vi "globalprogram.vi"() -> (2 "Array 2":i32[](array[numeric]), 3 "Numeric 2":i32)   [LabVIEW 2019]
uses:
  <vilib>/myRIO/Common/Instrument Driver Framework/Utilities/typedefs/Analog Scaling Constants.ctl
  <vilib>/myRIO/Common/Instrument Driver Framework/Utilities/typedefs/Analog Scaling Constants List.ctl
  <vilib>/myRIO/Common/Instrument Driver Framework/myRIO v1.0/AO/typedefs/AO Channels Enum.ctl
  <vilib>/myRIO/Common/Instrument Driver Framework/myRIO v1.0/AO/typedefs/AO Channels List.ctl
  <vilib>/myRIO/Common/Instrument Driver Framework/Utilities/typedefs/Generic FPGA Reference.ctl
  <vilib>/myRIO/Common/Instrument Driver Framework/Utilities/typedefs/myRIO v1.0 Reference.ctl
  <vilib>/myRIO/Common/Instrument Driver Framework/Utilities/typedefs/Hardware Version Enum.ctl
  <vilib>/myRIO/Common/Instrument Driver Framework/Utilities/typedefs/myRIO Generic Hardware Reference.ctl
  <vilib>/myRIO/Instrument Drivers/Onboard IO/AO/typedefs/AO Reference.ctl
  <vilib>/myRIO/Instrument Drivers/Onboard IO/AO/AO.lvlib
  <vilib>/myRIO/Instrument Drivers/Onboard IO/AO/vis/Write.vi
  <vilib>/userDefined/High Color/nirio_resource_hc.ctl
  <vilib>/myRIO/Common/Instrument Driver Framework/myRIO v1.0/AO/vis/myRIO v1.1 Open AO.vi
  <vilib>/myRIO/Instrument Drivers/Onboard IO/AO/vis/myRIO AO Open.xnode
  <vilib>/myRIO/Common/Instrument Driver Framework/Utilities/vis/Is FPGA Ref Available.vi
  <vilib>/myRIO/Express VI/Onboard IO/AO/AO Express VI.xnode
  Global 1.vi
  <vilib>/myRIO/Common/Instrument Driver Framework/myRIO v1.0/AI/typedefs/AI Channels Enum.ctl
  <vilib>/myRIO/Common/Instrument Driver Framework/myRIO v1.0/AI/typedefs/AI Channels List.ctl
  <vilib>/myRIO/Instrument Drivers/Onboard IO/AI/typedefs/AI Reference.ctl
  <vilib>/myRIO/Instrument Drivers/Onboard IO/AI/AI.lvlib
  <vilib>/myRIO/Instrument Drivers/Onboard IO/AI/vis/Read.vi
  <vilib>/myRIO/Common/Instrument Driver Framework/myRIO v1.0/AI/vis/myRIO v1.1 Open AI.vi
  <vilib>/myRIO/Instrument Drivers/Onboard IO/AI/vis/myRIO AI Open.xnode
  <vilib>/myRIO/Express VI/Onboard IO/AI/AI Express VI.xnode
  <vilib>/myRIO/Express VI/Onboard IO/DI/DI Express VI.xnode
  <vilib>/myRIO/Instrument Drivers/Onboard IO/DIO/vis/Read.vi
  <vilib>/myRIO/Instrument Drivers/Onboard IO/DIO/DIO.lvlib
  <vilib>/myRIO/Common/Instrument Driver Framework/myRIO v1.0/DIO/typedefs/DIO Channels Enum.ctl
  <vilib>/myRIO/Common/Instrument Driver Framework/myRIO v1.0/DIO/typedefs/DIO Channels List.ctl
  <vilib>/myRIO/Instrument Drivers/Onboard IO/DIO/typedefs/DIO Reference.ctl
  <vilib>/myRIO/Instrument Drivers/Onboard IO/DIO/vis/myRIO DIO Open.xnode
  <vilib>/myRIO/Instrument Drivers/Onboard IO/I2C/typedefs/I2C Transfer Rate.ctl
  <vilib>/myRIO/Instrument Drivers/Onboard IO/I2C/I2C.lvlib
  <vilib>/myRIO/Instrument Drivers/Onboard IO/I2C/typedefs/I2C User Configuration.ctl
  <vilib>/myRIO/Instrument Drivers/Onboard IO/I2C/typedefs/I2C Configuration.ctl
  <vilib>/myRIO/Common/Instrument Driver Framework/myRIO v1.0/I2C/typedefs/I2C Channels Enum.ctl
  <vilib>/myRIO/Instrument Drivers/Onboard IO/I2C/typedefs/I2C Reference.ctl
  <vilib>/myRIO/Instrument Drivers/Onboard IO/I2C/vis/Configure.vi
  <vilib>/myRIO/Instrument Drivers/Onboard IO/I2C/vis/Write.vi
  <vilib>/myRIO/Common/Instrument Driver Framework/myRIO v1.0/I2C/vis/myRIO v1.1 Open I2C.vi
  <vilib>/myRIO/Instrument Drivers/Onboard IO/I2C/vis/myRIO I2C Open.xnode
  <vilib>/myRIO/Express VI/Onboard IO/I2C/I2C Express VI.xnode
  <vilib>/myRIO/Common/Instrument Driver Framework/myRIO v1.0/DIO/vis/myRIO v1.1 Open DIO.vi
panel:
  in  "tijdsinterval 8":dbl
  in  "tijdsinterval 7":dbl
  in  "tijdsinterval 6":dbl
  in  "tijdsinterval 5":dbl
  in  "tijdsinterval 4":dbl
  in  "tijdsinterval 3":dbl
  in  "tijdsinterval 2":dbl
  out "groen":u32
  out "rood":u32
  out "error out 3":errorcluster
  in  "error in (no error) 3":errorcluster
  out "A/DIO1 (Pin 13)":bool
  in  "stoppen":bool
  in  "rechts draaien achteruit":bool
  in  "links draaien achteruit":bool
  out "appended array":dbl[](array[numeric])
  in  "snelheid":dbl
  in  "rechts draaien":bool
  in  "links draaien":bool
  in  "achterwaarts":bool
  in  "voorwaarts":bool
  in  "Boolean manueel":bool
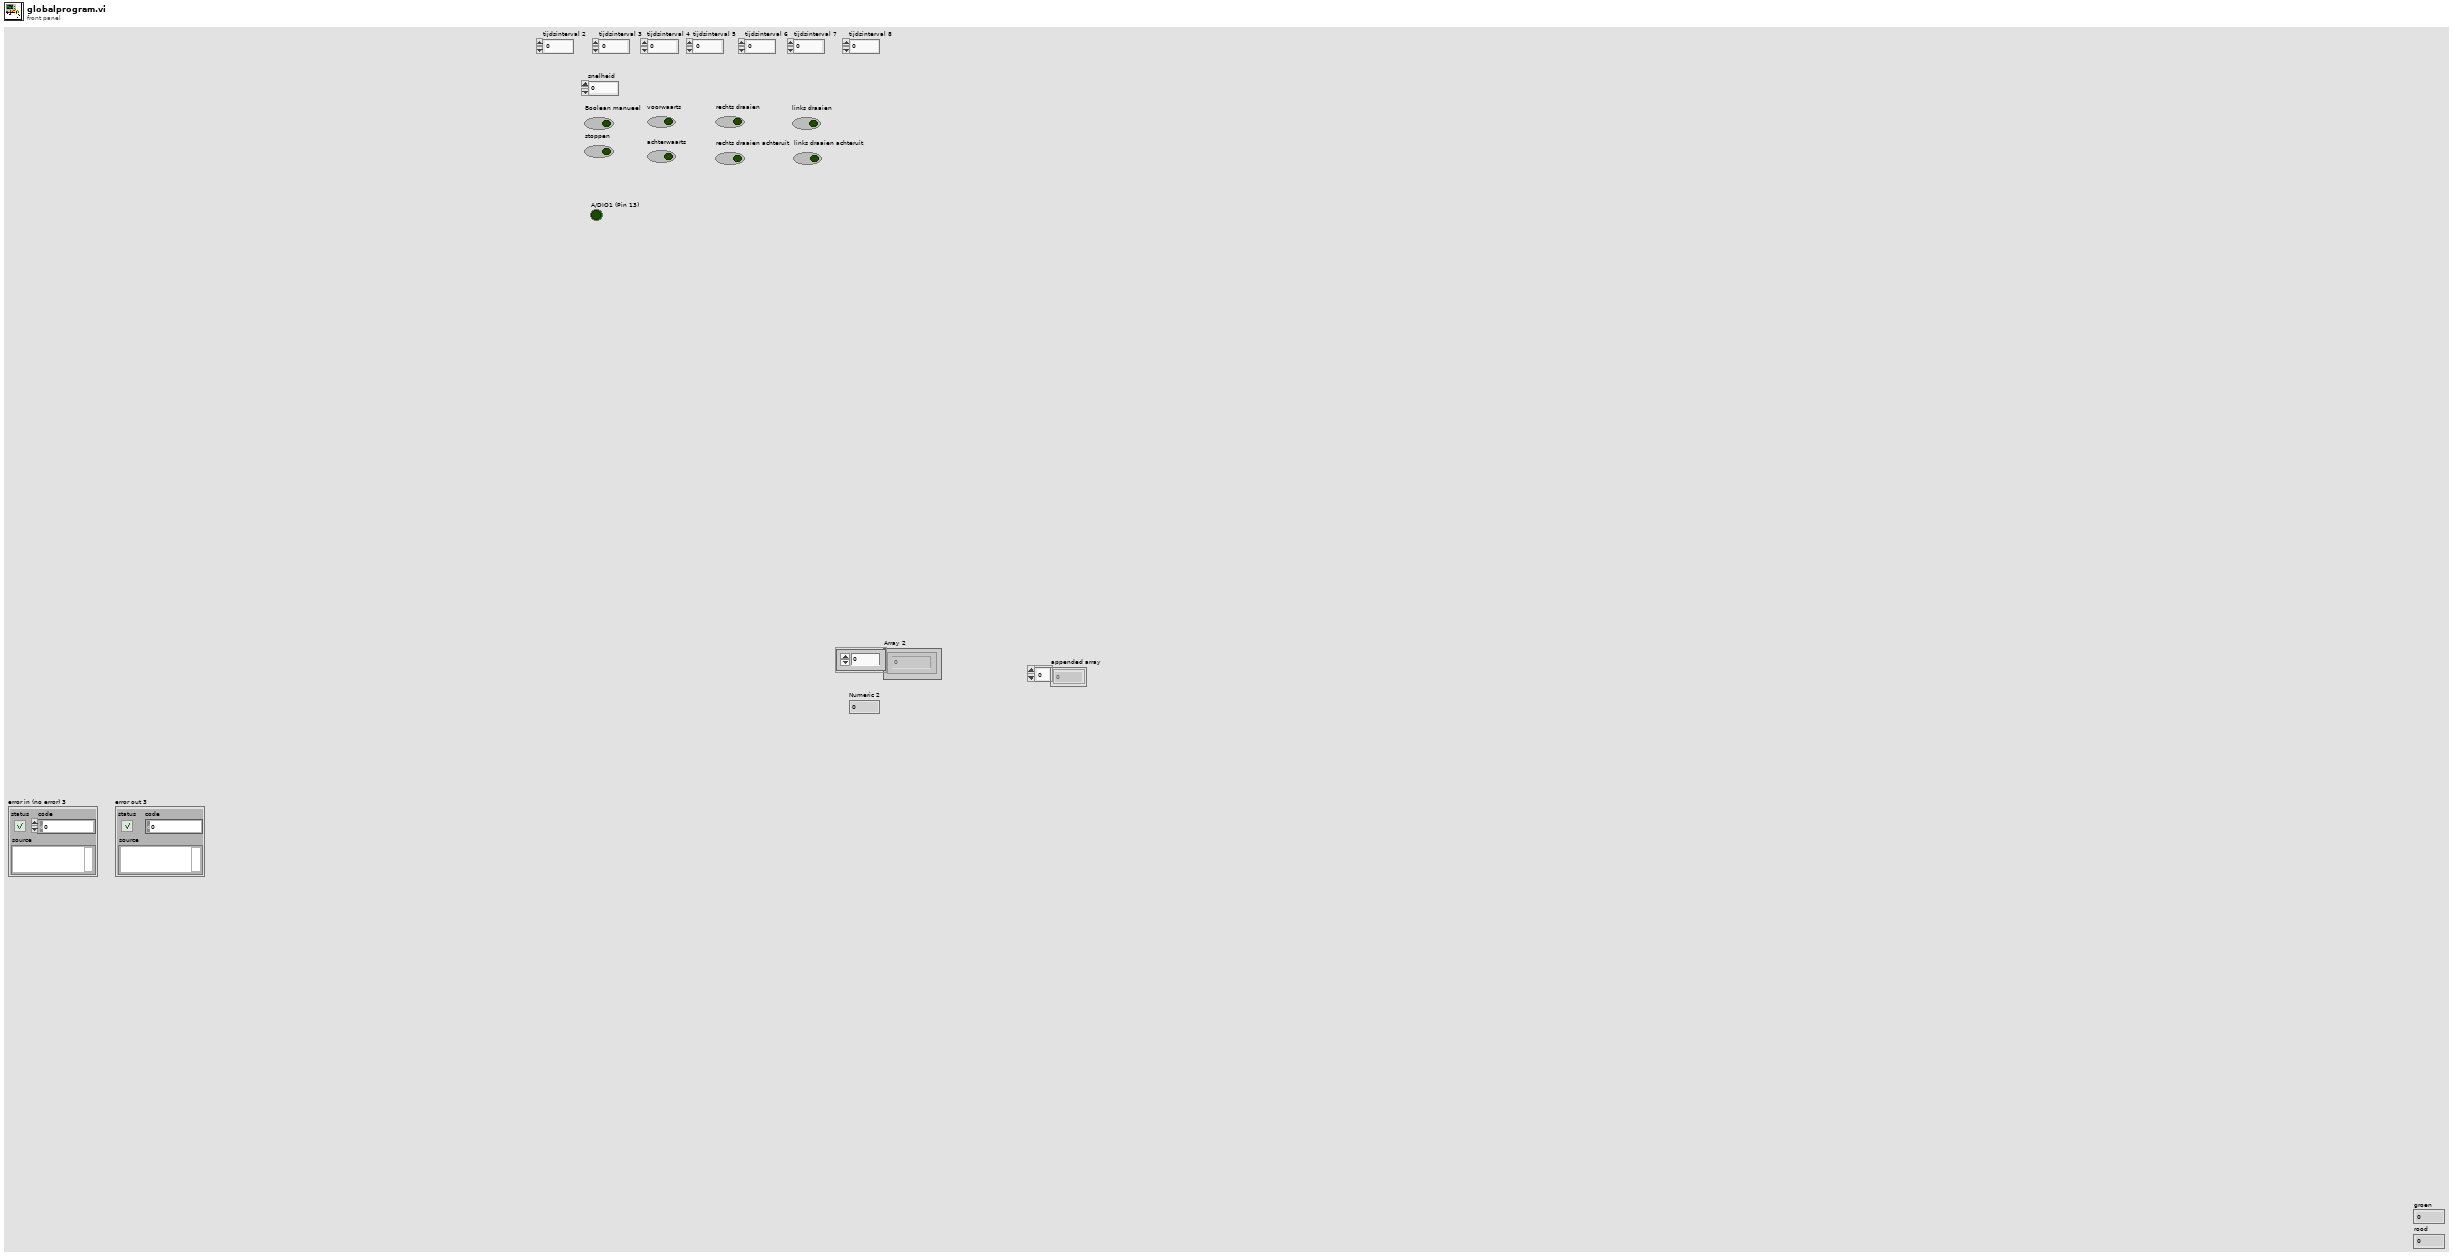
[diagram p1: front panel]
types:
  T1 = typedef "AO.lvlib/AO Reference.ctl" = cluster{"myRIO Reference":T2, "AO Channel List":T6, "AO Scaling Constant List":T8}
  T2 = typedef "myRIO Generic Hardware Reference.ctl" = cluster{"myRIO Model":T3, "myRIO Hardware Reference":T4}
  T3 = typedef "Hardware Version Enum.ctl" = enum16{"Unknown", "myRIO-1900", "myRIO-1950", "roboRIO", "NI ELVIS RIO CM", "ELVIS III"}
  T4 = typedef "myRIO v1.0 Reference.ctl" = cluster{"Generic FPGA Reference":T5, "Allow multiple opens":bool}
  T5 = typedef "Generic FPGA Reference.ctl" = refnum<k20>
  T6 = typedef "AO Channels List.ctl" = T7[]
  T7 = typedef "AO Channels Enum.ctl" = enum16{"Not Connected", "AudioOut/Left", "AudioOut/Right", "C/AO0", "C/AO1", "A/AO0", "A/AO1", "B/AO0", "B/AO1"}
  T8 = typedef "Analog Scaling Constants List.ctl" = T9[]
  T9 = typedef "Analog Scaling Constants.ctl" = cluster{"LSB Weight (Volts)":dbl, "Offset (Volts)":dbl, "Signed?":bool}
  T10 = typedef "nirio_resource_hc.ctl" = tag
  T11 = typedef "AI.lvlib/AI Reference.ctl" = cluster{"myRIO Reference":T2, "AI Channels List":T12, "AI Scaling Constants List":T8}
  T12 = typedef "AI Channels List.ctl" = T13[]
  T13 = typedef "AI Channels Enum.ctl" = enum16{"Not Connected", "AudioIn/Left", "AudioIn/Right", "C/AI0", "C/AI1", "A/AI0", "A/AI1", "A/AI2", "A/AI3", "A/AI4", "A/AI5", "A/AI6", "A/AI7", "B/AI0", "B/AI1", "B/AI2", "B/AI3", "B/AI4", "B/AI5", "B/AI6", "B/AI7", "AI/AI0", "AI/AI1", "AI/AI2", "AI/AI3", "A/AI0 (DIFF)", "A/AI1 (DIFF)", "A/AI2 (DIFF)", "A/AI3 (DIFF)", "B/AI0 (DIFF)", "B/AI1 (DIFF)", "B/AI2 (DIFF)", "B/AI3 (DIFF)"}
  T14 = typedef "I2C.lvlib/I2C Reference.ctl" = cluster{"myRIO Reference":T2, "I2C Channels Enum":T15, "I2C Configuration":T16}
  T15 = typedef "I2C Channels Enum.ctl" = enum16{"Not Connected", "A/I2C", "B/I2C", "I2C/I2C"}
  T16 = typedef "I2C.lvlib/I2C Configuration.ctl" = cluster{"I2C Transfer Rate":T17}
  T17 = typedef "I2C.lvlib/I2C Transfer Rate.ctl" = enum16{"Standard mode (100 kbps)", "Fast mode (400 kbps)"}
  T18 = typedef "I2C.lvlib/I2C User Configuration.ctl" = cluster{"I2C Transfer Rate":T17}
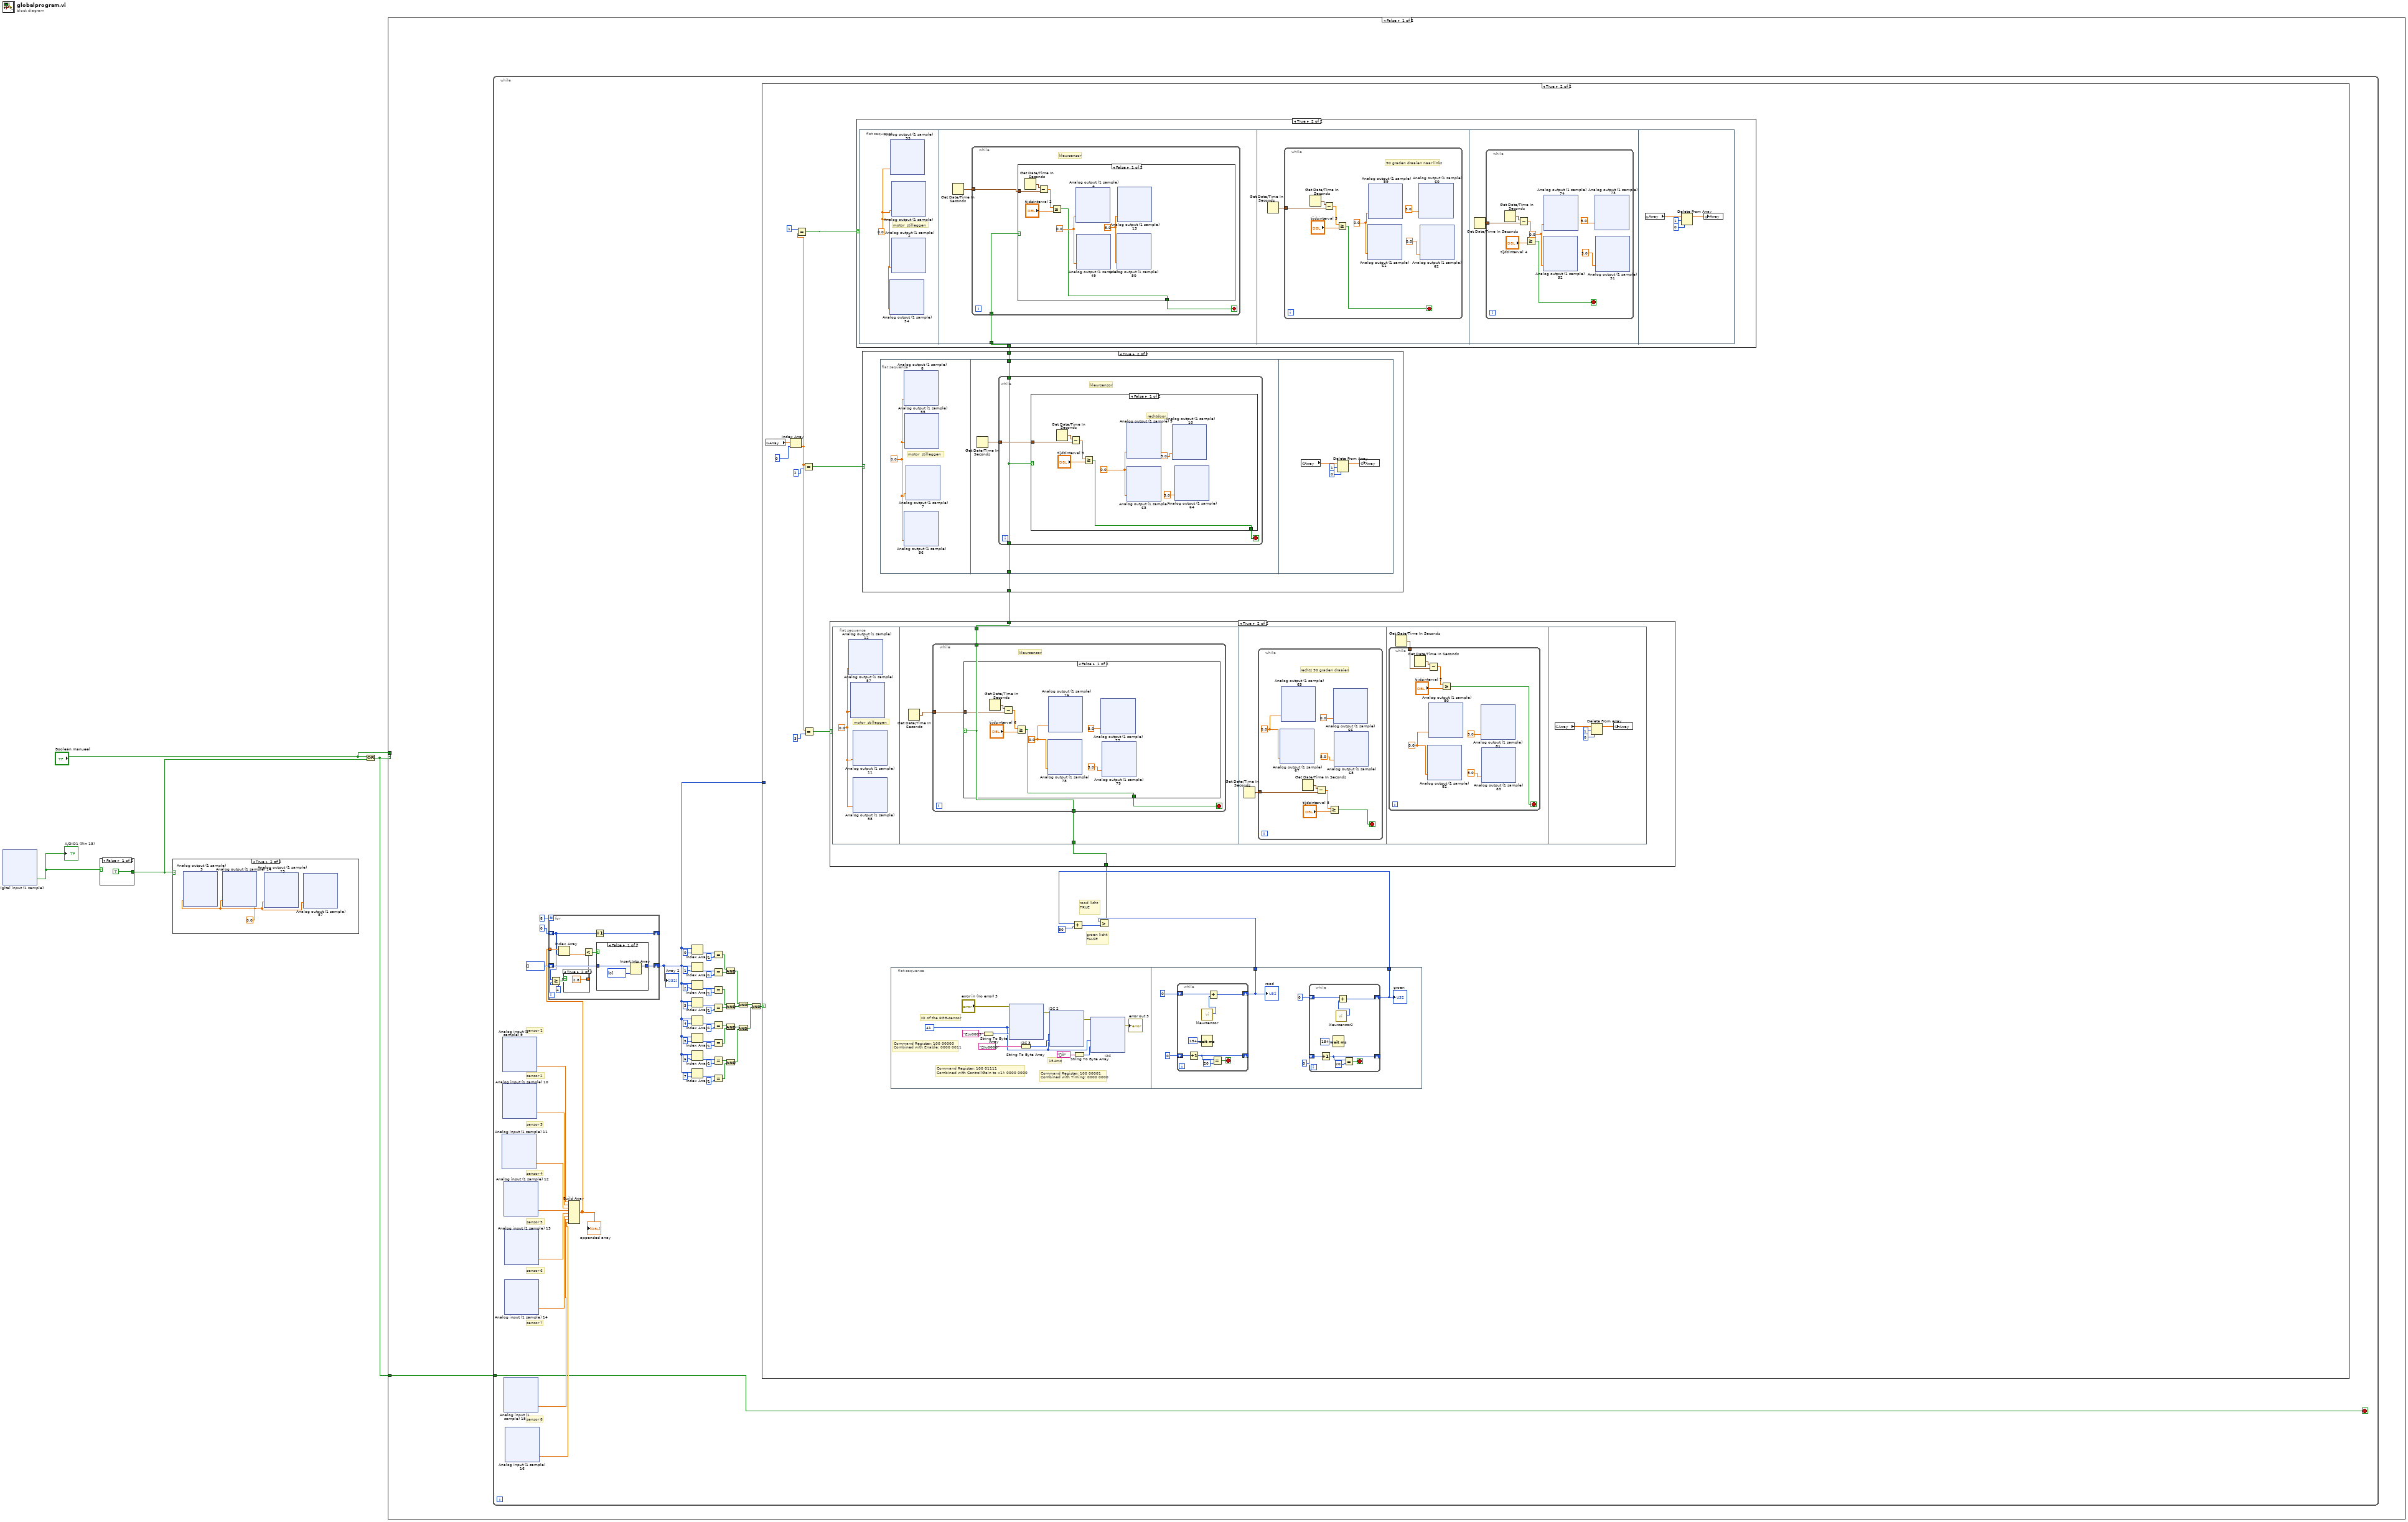
[diagram p0: block diagram]
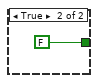
[diagram p2: hidden frame]
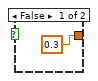
[diagram p4: hidden frame]
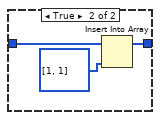
[diagram p5: hidden frame]
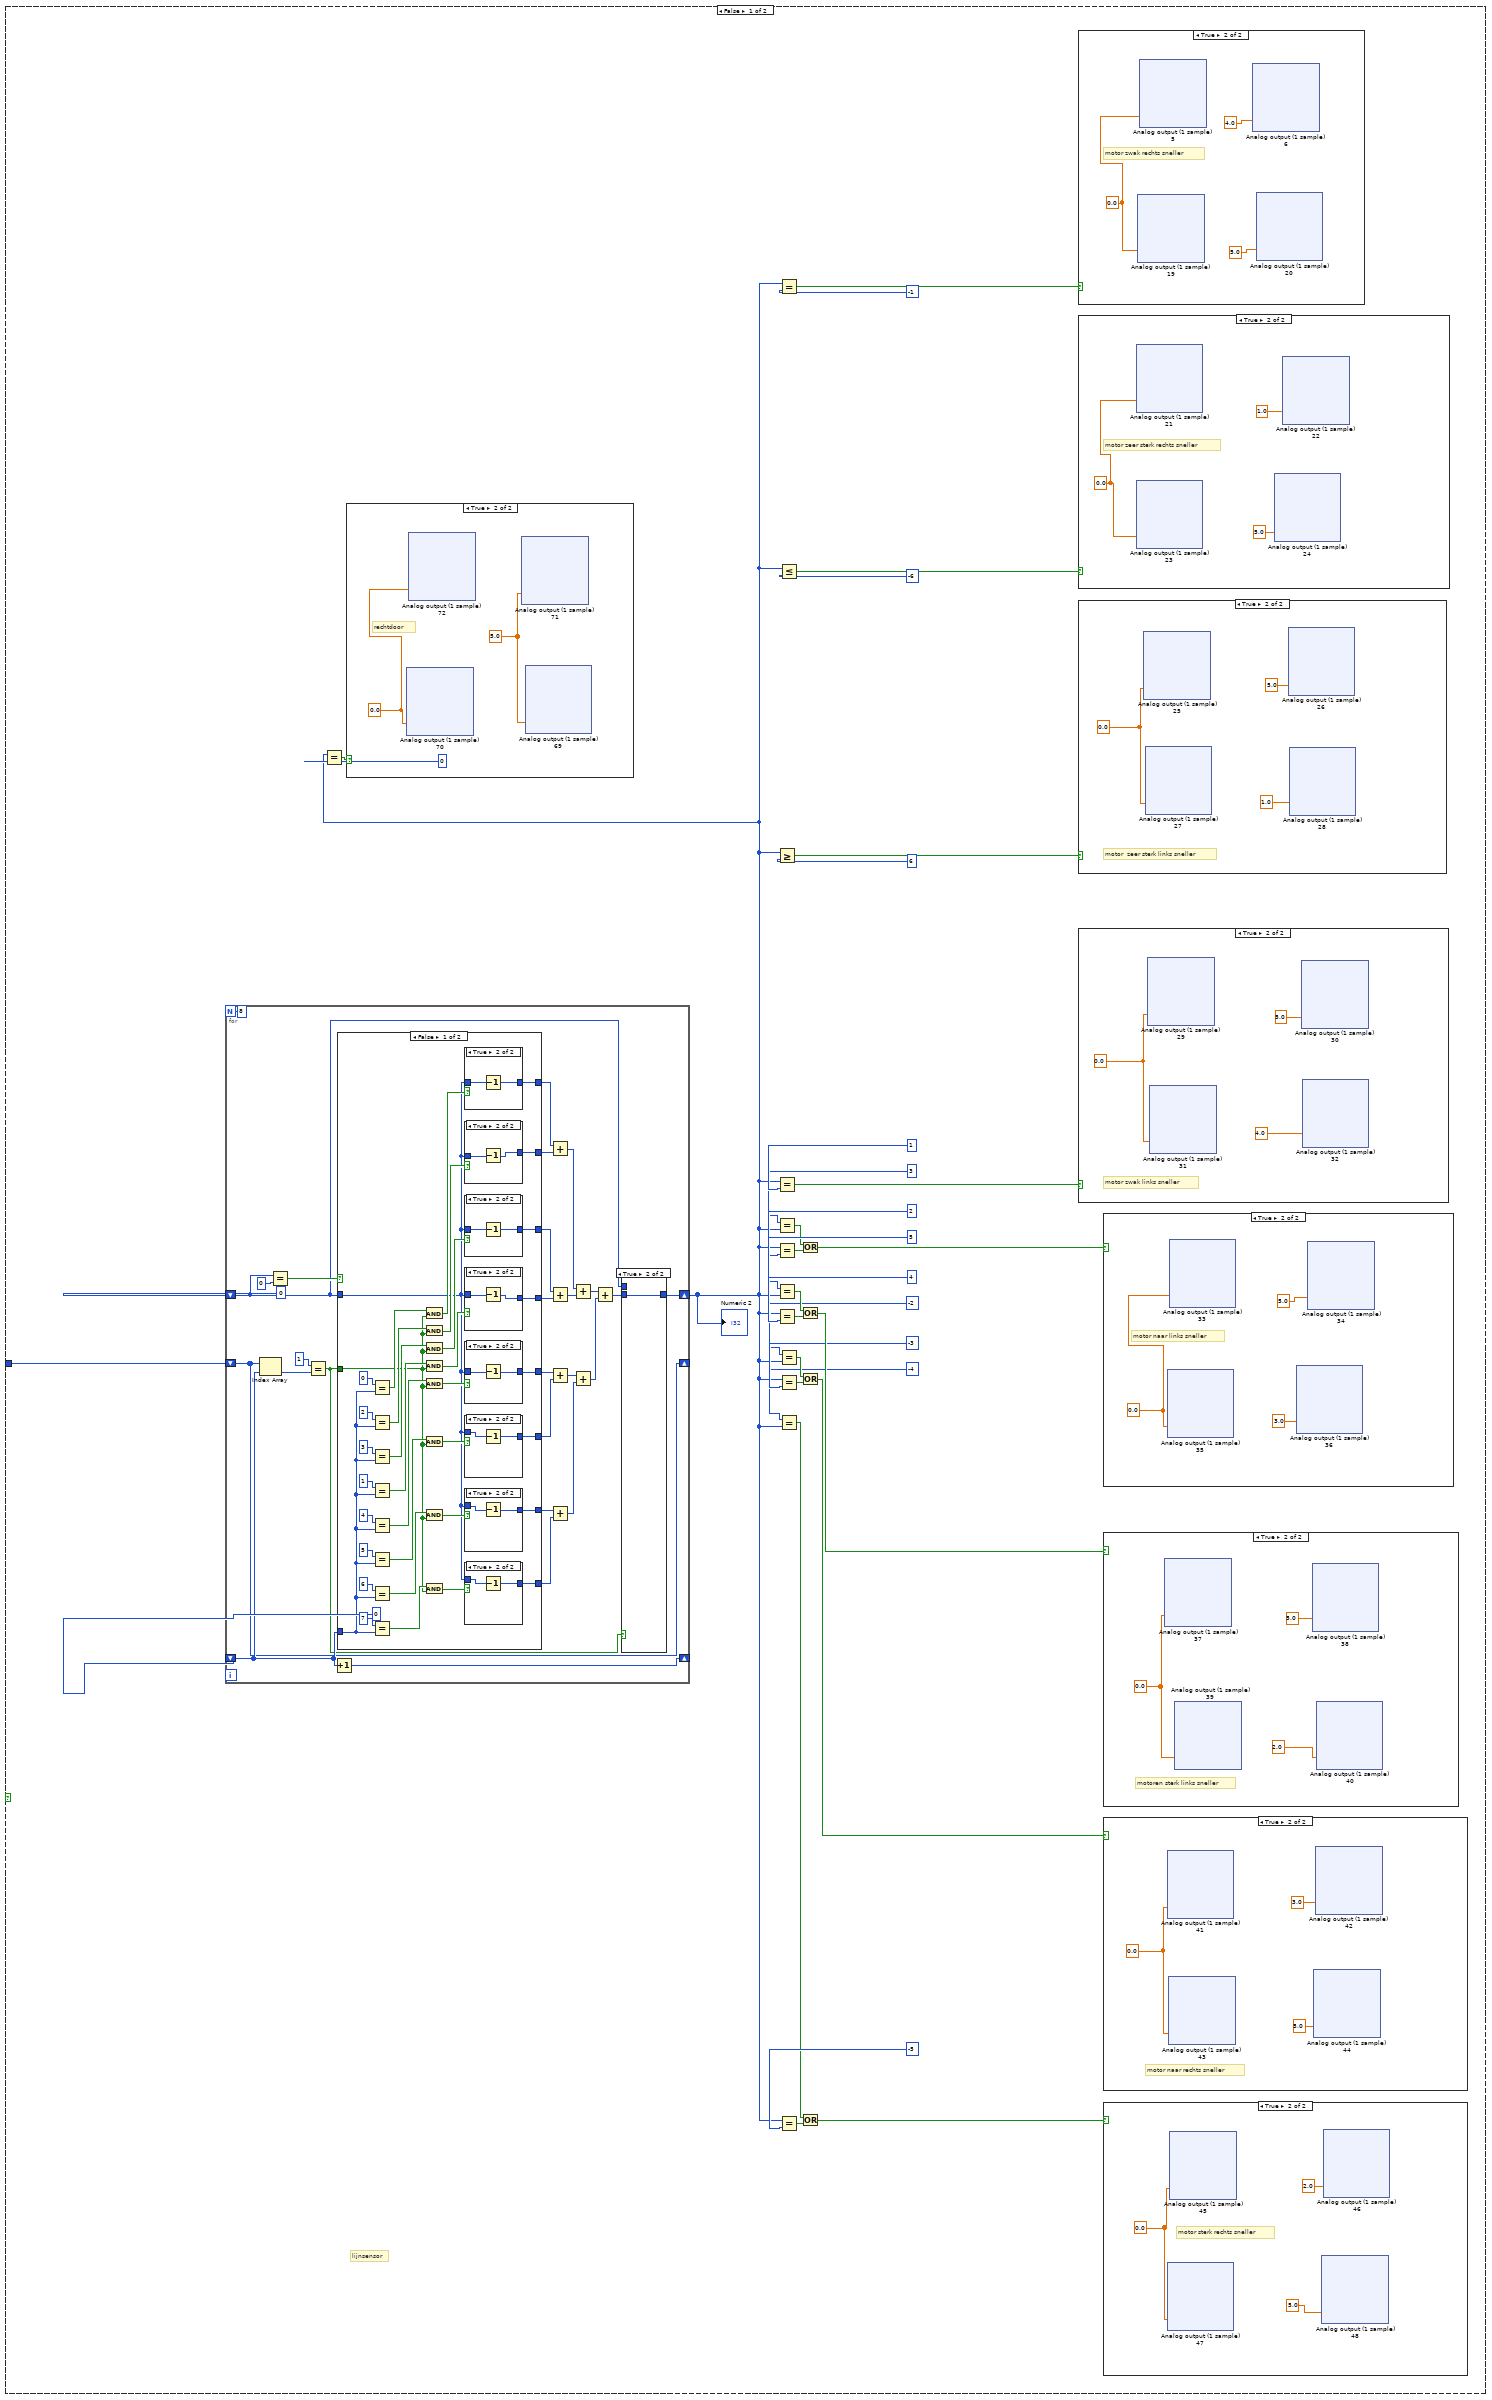
[diagram p6: hidden frame]
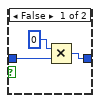
[diagram p17: hidden frame]
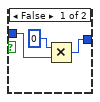
[diagram p18: hidden frame]
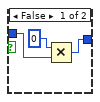
[diagram p19: hidden frame]
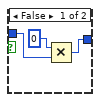
[diagram p20: hidden frame]
diagram:
  n1 = xnode "Digital input (1 sample)"() -> ("A/DIO1 (Pin 13)"=w1:bool)  [unwired: 1 in, 1 out]
  "A/DIO1 (Pin 13)" <- w1
  n2 = case shown="False" w1 {
    tunnel: [TRUE FALSE] -> w2
    frame False {
    }
    frame True {
    }
  }
  n3 = case shown="True" w2 {
    frame False {
    }
    frame True {
      w7 = 0.0
      n4 = xnode "Analog output (1 sample) 3"("A/AO0 (Pin 2)"=w7) -> ()  [unwired: 1 in, 1 out]
      n5 = xnode "Analog output (1 sample) 14"("A/AO1 (Pin 4)"=w7) -> ()  [unwired: 1 in, 1 out]
      n6 = xnode "Analog output (1 sample) 75"("B/AO0 (Pin 2)"=w7) -> ()  [unwired: 1 in, 1 out]
      n7 = xnode "Analog output (1 sample) 87"("B/AO1 (Pin 4)"=w7) -> ()  [unwired: 1 in, 1 out]
    }
  }
  n8 = Or(x="Boolean manueel", y=w2) -> (x .or. y?=w4:bool)
  n9 = case shown="False" w4 {
    tunnel: w4 -> [w156 _]
    tunnel: "Boolean manueel" -> [_ w3844]
    frame False {
      n10 = while {
        tunnel: w156 -> [w157]
        stop <- w157 stop-if-true
        # "sensor 8"
        # "sensor 7"
        # "sensor 6"
        # "sensor 5"
        # "sensor 4"
        # "sensor 3"
        # "sensor 2"
        # "sensor 1"
        n11 = xnode "Analog input (1 sample) 11"() -> ("A/AI1 (Pin 5)"=w164:dbl)  [unwired: 1 in, 1 out]
        n12 = xnode "Analog input (1 sample) 9"() -> ("A/AI3 (Pin 9)"=w166:dbl)  [unwired: 1 in, 1 out]
        n13 = xnode "Analog input (1 sample) 10"() -> ("A/AI2 (Pin 7)"=w165:dbl)  [unwired: 1 in, 1 out]
        n14 = xnode "Analog input (1 sample) 12"() -> ("A/AI0 (Pin 3)"=w163:dbl)  [unwired: 1 in, 1 out]
        n15 = xnode "Analog input (1 sample) 15"() -> ("A/AI1 (Pin 5)"=w160:dbl)  [unwired: 1 in, 1 out]
        n16 = xnode "Analog input (1 sample) 14"() -> ("B/AI2 (Pin 7)"=w161:dbl)  [unwired: 1 in, 1 out]
        n17 = xnode "Analog input (1 sample) 13"() -> ("B/AI3 (Pin 9)"=w162:dbl)  [unwired: 1 in, 1 out]
        n18 = xnode "Analog input (1 sample) 16"() -> ("B/AI0 (Pin 3)"=w159:dbl)  [unwired: 1 in, 1 out]
        n19 = Build Array(w166, w165, w164, w163, w162, w161, w160, w159) -> (w158:dbl[])
        "appended array" <- w158
        n20 = for {
          N: 8 -> [_]
          shift-right: [w514] -> w209
          shift-left: i32[] [] -> [w515]
          shift-right: [w512] -> _
          shift-left: 0 -> [w507]
          tunnel: w158 -> [w510]
          n21 = Greater Or Equal?(x=w507, y=4) -> (x >= y?=w508:bool)
          n22 = Index Array(array=w510, index=w507) -> (element=w511:dbl)
          n23 = case shown="True" w508 {
            tunnel: [0.3 2.8] -> w509
            frame False {
            }
            frame True {
            }
          }
          n24 = Less?(x=w509, y=w511) -> (x < y?=w513:bool)
          n25 = Increment(x=w507) -> (x+1=w512:i32)
          n26 = case shown="False" w513 {
            tunnel: w515 -> [w519 w521]
            tunnel: [w520 w523] -> w514
            frame False {
              n27 = Insert Into Array(array=w519, new element=i32[] [0]) -> (w520:i32[])  [unwired: 1 in]
            }
            frame True {
              n28 = Insert Into Array(array=w521, new element=i32[] [1, 1]) -> (w523:i32[])  [unwired: 1 in]
            }
          }
        }
        "Array 2" <- w209
        n29 = Index Array(array=w209, index=0) -> (element=w188:i32)
        n30 = Index Array(array=w209, index=1) -> (element=w167:i32)
        n31 = Index Array(array=w209, index=2) -> (element=w173:i32)
        n32 = Index Array(array=w209, index=3) -> (element=w170:i32)
        n33 = Index Array(array=w209, index=4) -> (element=w176:i32)
        n34 = Index Array(array=w209, index=5) -> (element=w179:i32)
        n35 = Index Array(array=w209, index=6) -> (element=w182:i32)
        n36 = Index Array(array=w209, index=7) -> (element=w185:i32)
        n37 = Equal?(x=w188, y=1) -> (x = y?=w191:bool)
        n38 = Equal?(x=w167, y=1) -> (x = y?=w192:bool)
        n39 = Equal?(x=w173, y=1) -> (x = y?=w193:bool)
        n40 = Equal?(x=w170, y=1) -> (x = y?=w194:bool)
        n41 = Equal?(x=w176, y=1) -> (x = y?=w195:bool)
        n42 = Equal?(x=w179, y=1) -> (x = y?=w196:bool)
        n43 = Equal?(x=w182, y=1) -> (x = y?=w197:bool)
        n44 = Equal?(x=w185, y=1) -> (x = y?=w198:bool)
        n45 = And(x=w191, y=w192) -> (x .and. y?=w199:bool)
        n46 = And(x=w193, y=w194) -> (x .and. y?=w200:bool)
        n47 = And(x=w195, y=w196) -> (x .and. y?=w201:bool)
        n48 = And(x=w197, y=w198) -> (x .and. y?=w202:bool)
        n49 = And(x=w199, y=w200) -> (x .and. y?=w203:bool)
        n50 = And(x=w201, y=w202) -> (x .and. y?=w204:bool)
        n51 = And(x=w203, y=w204) -> (x .and. y?=w205:bool)
        n52 = case shown="True" w205 {
          tunnel: w209 -> [w527 _]
          frame False {
            # "lijnsensor"
            n53 = for {
              N: 8 -> [_]
              shift-right: [w1927] -> _
              shift-left: 0 -> [w1941]
              shift-right: [w1919] -> w524
              shift-left: 0 -> [w1920]
              shift-right: [w1932] -> _
              shift-left: w527 -> [w1932]
              n54 = Index Array(array=w1932, index=w1941) -> (element=w1931:i32)
              n55 = Equal?(x=w1920, y=0) -> (x = y?=w1928:bool)
              n56 = Equal?(x=1, y=w1931) -> (x = y?=w1918:bool)
              n57 = Increment(x=w1941) -> (x+1=w1927:i32)
              n58 = case shown="False" w1928 {
                tunnel: w1941 -> [w1951 w2037]
                tunnel: [w1945 w2036] -> w1940
                tunnel: [w1952 w2035] -> w1939
                tunnel: [w1953 w2034] -> w1938
                tunnel: [w1954 w2033] -> w1937
                tunnel: w1920 -> [w1944 w2032]
                tunnel: w1918 -> [w1950 w2023]
                tunnel: [w1948 w2022] -> w1926
                tunnel: [w1949 w2021] -> w1925
                tunnel: [w1946 w2020] -> w1923
                tunnel: [w1947 w2019] -> w1922
                frame False {
                  n59 = Equal?(x=0, y=w1951) -> (x = y?=w1971:bool)
                  n60 = Equal?(x=2, y=w1951) -> (x = y?=w1977:bool)
                  n61 = Equal?(x=3, y=w1951) -> (x = y?=w1978:bool)
                  n62 = Equal?(x=1, y=w1951) -> (x = y?=w1963:bool)
                  n63 = Equal?(x=4, y=w1951) -> (x = y?=w1975:bool)
                  n64 = Equal?(x=5, y=w1951) -> (x = y?=w1976:bool)
                  n65 = Equal?(x=6, y=w1951) -> (x = y?=w1974:bool)
                  n66 = Equal?(x=7, y=w1951) -> (x = y?=w1973:bool)
                  n67 = And(x=w1971, y=w1950) -> (x .and. y?=w1955:bool)
                  n68 = And(x=w1977, y=w1950) -> (x .and. y?=w1957:bool)
                  n69 = And(x=w1978, y=w1950) -> (x .and. y?=w1958:bool)
                  n70 = And(x=w1963, y=w1950) -> (x .and. y?=w1956:bool)
                  n71 = And(x=w1975, y=w1950) -> (x .and. y?=w1959:bool)
                  n72 = And(x=w1976, y=w1950) -> (x .and. y?=w1960:bool)
                  n73 = And(x=w1974, y=w1950) -> (x .and. y?=w1961:bool)
                  n74 = And(x=w1973, y=w1950) -> (x .and. y?=w1962:bool)
                  n75 = case shown="True" w1955 {
                    tunnel: [w1980 w1983] -> w1949
                    tunnel: w1944 -> [w1979 w1982]
                    frame False {
                      n76 = Multiply(x=0, y=w1979) -> (x*y=w1980:i32)
                    }
                    frame True {
                      n77 = Decrement(x=w1982) -> (x-1=w1983:i32)
                    }
                  }
                  n78 = case shown="True" w1957 {
                    tunnel: [w2011 w2012] -> w1948
                    tunnel: w1944 -> [w2010 w2013]
                    frame False {
                      n79 = Multiply(x=0, y=w2010) -> (x*y=w2011:i32)
                    }
                    frame True {
                      n80 = Decrement(x=w2013) -> (x-1=w2012:i32)
                    }
                  }
                  n81 = case shown="True" w1958 {
                    tunnel: [w2005 w2008] -> w1947
                    tunnel: w1944 -> [w2004 w2007]
                    frame False {
                      n82 = Multiply(x=0, y=w2004) -> (x*y=w2005:i32)
                    }
                    frame True {
                      n83 = Decrement(x=w2007) -> (x-1=w2008:i32)
                    }
                  }
                  n84 = case shown="True" w1956 {
                    tunnel: [w2015 w2018] -> w1946
                    tunnel: w1944 -> [w2014 w2017]
                    frame False {
                      n85 = Multiply(x=0, y=w2014) -> (x*y=w2015:i32)
                    }
                    frame True {
                      n86 = Decrement(x=w2017) -> (x-1=w2018:i32)
                    }
                  }
                  n87 = case shown="True" w1959 {
                    tunnel: [w2000 w2003] -> w1945
                    tunnel: w1944 -> [w1999 w2002]
                    frame False {
                      n88 = Multiply(x=0, y=w1999) -> (x*y=w2000:i32)
                    }
                    frame True {
                      n89 = Decrement(x=w2002) -> (x-1=w2003:i32)
                    }
                  }
                  n90 = case shown="True" w1960 {
                    tunnel: [w1990 w1993] -> w1952
                    tunnel: w1944 -> [w1989 w1992]
                    frame False {
                      n91 = Multiply(x=0, y=w1989) -> (x*y=w1990:i32)
                    }
                    frame True {
                      n92 = Decrement(x=w1992) -> (x-1=w1993:i32)
                    }
                  }
                  n93 = case shown="True" w1961 {
                    tunnel: [w1995 w1998] -> w1953
                    tunnel: w1944 -> [w1994 w1997]
                    frame False {
                      n94 = Multiply(x=0, y=w1994) -> (x*y=w1995:i32)
                    }
                    frame True {
                      n95 = Decrement(x=w1997) -> (x-1=w1998:i32)
                    }
                  }
                  n96 = case shown="True" w1962 {
                    tunnel: [w1984 w1988] -> w1954
                    tunnel: w1944 -> [w1985 w1987]
                    frame False {
                      n97 = Multiply(x=0, y=w1985) -> (x*y=w1984:i32)
                    }
                    frame True {
                      n98 = Decrement(x=w1987) -> (x-1=w1988:i32)
                    }
                  }
                }
                frame True {
                  n99 = Equal?(x=0, y=w2037) -> (x = y?=w2046:bool)
                  n100 = Equal?(x=1, y=w2037) -> (x = y?=w2038:bool)
                  n101 = Equal?(x=2, y=w2037) -> (x = y?=w2052:bool)
                  n102 = Equal?(x=3, y=w2037) -> (x = y?=w2053:bool)
                  n103 = Equal?(x=4, y=w2037) -> (x = y?=w2050:bool)
                  n104 = Equal?(x=5, y=w2037) -> (x = y?=w2051:bool)
                  n105 = Equal?(x=6, y=w2037) -> (x = y?=w2049:bool)
                  n106 = Equal?(x=7, y=w2037) -> (x = y?=w2048:bool)
                  n107 = And(x=w2046, y=w2023) -> (x .and. y?=w2024:bool)
                  n108 = And(x=w2038, y=w2023) -> (x .and. y?=w2025:bool)
                  n109 = And(x=w2052, y=w2023) -> (x .and. y?=w2026:bool)
                  n110 = And(x=w2053, y=w2023) -> (x .and. y?=w2027:bool)
                  n111 = And(x=w2050, y=w2023) -> (x .and. y?=w2028:bool)
                  n112 = And(x=w2051, y=w2023) -> (x .and. y?=w2029:bool)
                  n113 = And(x=w2049, y=w2023) -> (x .and. y?=w2030:bool)
                  n114 = And(x=w2048, y=w2023) -> (x .and. y?=w2031:bool)
                  n115 = case shown="True" w2024 {
                    tunnel: w2032 -> [w2054 w2058]
                    tunnel: [w2055 w2057] -> w2021
                    frame False {
                      n116 = Multiply(x=0, y=w2054) -> (x*y=w2055:i32)
                    }
                    frame True {
                      n117 = Add(x=7, y=w2058) -> (x+y=w2057:i32)
                    }
                  }
                  n118 = case shown="True" w2025 {
                    tunnel: w2032 -> [w2094 w2097]
                    tunnel: [w2095 w2098] -> w2022
                    frame False {
                      n119 = Multiply(x=0, y=w2094) -> (x*y=w2095:i32)
                    }
                    frame True {
                      n120 = Add(x=5, y=w2097) -> (x+y=w2098:i32)
                    }
                  }
                  n121 = case shown="True" w2026 {
                    tunnel: w2032 -> [w2088 w2092]
                    tunnel: [w2089 w2091] -> w2019
                    frame False {
                      n122 = Multiply(x=0, y=w2088) -> (x*y=w2089:i32)
                    }
                    frame True {
                      n123 = Add(x=3, y=w2092) -> (x+y=w2091:i32)
                    }
                  }
                  n124 = case shown="True" w2027 {
                    tunnel: w2032 -> [w2084 w2087]
                    tunnel: [w2083 w2086] -> w2020
                    frame False {
                      n125 = Multiply(x=0, y=w2084) -> (x*y=w2083:i32)
                    }
                    frame True {
                      n126 = Increment(x=w2087) -> (x+1=w2086:i32)
                    }
                  }
                  n127 = case shown="True" w2028 {
                    tunnel: w2032 -> [w2078 w2082]
                    tunnel: [w2079 w2081] -> w2036
                    frame False {
                      n128 = Multiply(x=0, y=w2078) -> (x*y=w2079:i32)
                    }
                    frame True {
                      n129 = Decrement(x=w2082) -> (x-1=w2081:i32)
                    }
                  }
                  n130 = case shown="True" w2029 {
                    tunnel: w2032 -> [w2067 w2069]
                    tunnel: [w2066 w2071] -> w2035
                    frame False {
                      n131 = Multiply(x=0, y=w2067) -> (x*y=w2066:i32)
                    }
                    frame True {
                      n132 = Subtract(x=w2069, y=3) -> (x-y=w2071:i32)
                    }
                  }
                  n133 = case shown="True" w2030 {
                    tunnel: w2032 -> [w2073 w2075]
                    tunnel: [w2072 w2076] -> w2034
                    frame False {
                      n134 = Multiply(x=0, y=w2073) -> (x*y=w2072:i32)
                    }
                    frame True {
                      n135 = Subtract(x=w2075, y=5) -> (x-y=w2076:i32)
                    }
                  }
                  n136 = case shown="True" w2031 {
                    tunnel: w2032 -> [w2060 w2063]
                    tunnel: [w2061 w2064] -> w2033
                    frame False {
                      n137 = Multiply(x=0, y=w2060) -> (x*y=w2061:i32)
                    }
                    frame True {
                      n138 = Subtract(x=w2063, y=7) -> (x-y=w2064:i32)
                    }
                  }
                }
              }
              n139 = Add(x=w1925, y=w1926) -> (x+y=w1924:i32)
              n140 = Add(x=w1922, y=w1923) -> (x+y=w1921:i32)
              n141 = Add(x=w1940, y=w1939) -> (x+y=w1935:i32)
              n142 = Add(x=w1938, y=w1937) -> (x+y=w1936:i32)
              n143 = Add(x=w1924, y=w1921) -> (x+y=w1934:i32)
              n144 = Add(x=w1935, y=w1936) -> (x+y=w1933:i32)
              n145 = Add(x=w1934, y=w1933) -> (x+y=w1917:i32)
              n146 = case shown="True" w1918 {
                tunnel: w1920 -> [w1942 _]
                tunnel: [w1942 w1943] -> w1919
                tunnel: w1917 -> [_ w1943]
                frame False {
                }
                frame True {
                }
              }
            }
            "Numeric 2" <- w524
            n147 = Equal?(x=w524, y=0) -> (x = y?=w525:bool)
            n148 = case shown="True" w525 {
              frame False {
              }
              frame True {
                w560 = 5.0
                w559 = 0.0
                # "rechtdoor"
                n149 = xnode "Analog output (1 sample) 70"("B/AO0 (Pin 2)"=w559) -> ()  [unwired: 1 in, 1 out]
                n150 = xnode "Analog output (1 sample) 72"("A/AO0 (Pin 2)"=w559) -> ()  [unwired: 1 in, 1 out]
                n151 = xnode "Analog output (1 sample) 71"("A/AO1 (Pin 4)"=w560) -> ()  [unwired: 1 in, 1 out]
                n152 = xnode "Analog output (1 sample) 69"("B/AO1 (Pin 4)"=w560) -> ()  [unwired: 1 in, 1 out]
              }
            }
            n153 = Greater Or Equal?(x=w524, y=6) -> (x >= y?=w553:bool)
            n154 = Equal?(x=w524, y=1) -> (x = y?=w554:bool)
            n155 = Equal?(x=3, y=w524) -> (x = y?=w544:bool)
            n156 = Equal?(x=w524, y=2) -> (x = y?=w545:bool)
            n157 = Equal?(x=5, y=w524) -> (x = y?=w548:bool)
            n158 = Equal?(x=w524, y=4) -> (x = y?=w549:bool)
            n159 = Equal?(x=w524, y=-1) -> (x = y?=w532:bool)
            n160 = Less Or Equal?(x=w524, y=-6) -> (x <= y?=w530:bool)
            n161 = Equal?(x=-2, y=w524) -> (x = y?=w538:bool)
            n162 = Equal?(x=w524, y=-3) -> (x = y?=w539:bool)
            n163 = Equal?(x=-4, y=w524) -> (x = y?=w534:bool)
            n164 = Equal?(x=w524, y=-5) -> (x = y?=w535:bool)
            n165 = Or(x=w544, y=w545) -> (x .or. y?=w542:bool)
            n166 = Or(x=w548, y=w549) -> (x .or. y?=w550:bool)
            n167 = Or(x=w538, y=w539) -> (x .or. y?=w531:bool)
            n168 = Or(x=w534, y=w535) -> (x .or. y?=w528:bool)
            n169 = case shown="True" w532 {
              frame False {
              }
              frame True {
                w1466 = 0.0
                # "motor zwak rechts sneller"
                n170 = xnode "Analog output (1 sample) 19"("B/AO0 (Pin 2)"=w1466) -> ()  [unwired: 1 in, 1 out]
                n171 = xnode "Analog output (1 sample) 5"("A/AO0 (Pin 2)"=w1466) -> ()  [unwired: 1 in, 1 out]
                n172 = xnode "Analog output (1 sample) 6"("A/AO1 (Pin 4)"=4.0) -> ()  [unwired: 1 in, 1 out]
                n173 = xnode "Analog output (1 sample) 20"("B/AO1 (Pin 4)"=5.0) -> ()  [unwired: 1 in, 1 out]
              }
            }
            n174 = case shown="True" w530 {
              frame False {
              }
              frame True {
                w1013 = 0.0
                # "motor zeer sterk rechts sneller"
                n175 = xnode "Analog output (1 sample) 21"("A/AO0 (Pin 2)"=w1013) -> ()  [unwired: 1 in, 1 out]
                n176 = xnode "Analog output (1 sample) 23"("B/AO0 (Pin 2)"=w1013) -> ()  [unwired: 1 in, 1 out]
                n177 = xnode "Analog output (1 sample) 24"("B/AO1 (Pin 4)"=5.0) -> ()  [unwired: 1 in, 1 out]
                n178 = xnode "Analog output (1 sample) 22"("A/AO1 (Pin 4)"=1.0) -> ()  [unwired: 1 in, 1 out]
              }
            }
            n179 = case shown="True" w553 {
              frame False {
              }
              frame True {
                w1768 = 0.0
                # "motor  zeer sterk links sneller"
                n180 = xnode "Analog output (1 sample) 25"("A/AO0 (Pin 2)"=w1768) -> ()  [unwired: 1 in, 1 out]
                n181 = xnode "Analog output (1 sample) 27"("B/AO0 (Pin 2)"=w1768) -> ()  [unwired: 1 in, 1 out]
                n182 = xnode "Analog output (1 sample) 26"("A/AO1 (Pin 4)"=5.0) -> ()  [unwired: 1 in, 1 out]
                n183 = xnode "Analog output (1 sample) 28"("B/AO1 (Pin 4)"=1.0) -> ()  [unwired: 1 in, 1 out]
              }
            }
            n184 = case shown="True" w554 {
              frame False {
              }
              frame True {
                w862 = 0.0
                # "motor zwak links sneller"
                n185 = xnode "Analog output (1 sample) 29"("A/AO0 (Pin 2)"=w862) -> ()  [unwired: 1 in, 1 out]
                n186 = xnode "Analog output (1 sample) 31"("B/AO0 (Pin 2)"=w862) -> ()  [unwired: 1 in, 1 out]
                n187 = xnode "Analog output (1 sample) 30"("A/AO1 (Pin 4)"=5.0) -> ()  [unwired: 1 in, 1 out]
                n188 = xnode "Analog output (1 sample) 32"("B/AO1 (Pin 4)"=4.0) -> ()  [unwired: 1 in, 1 out]
              }
            }
            n189 = case shown="True" w542 {
              frame False {
              }
              frame True {
                w1164 = 0.0
                # "motor naar links sneller"
                n190 = xnode "Analog output (1 sample) 35"("B/AO0 (Pin 2)"=w1164) -> ()  [unwired: 1 in, 1 out]
                n191 = xnode "Analog output (1 sample) 33"("A/AO0 (Pin 2)"=w1164) -> ()  [unwired: 1 in, 1 out]
                n192 = xnode "Analog output (1 sample) 36"("B/AO1 (Pin 4)"=3.0) -> ()  [unwired: 1 in, 1 out]
                n193 = xnode "Analog output (1 sample) 34"("A/AO1 (Pin 4)"=5.0) -> ()  [unwired: 1 in, 1 out]
              }
            }
            n194 = case shown="True" w550 {
              frame False {
              }
              frame True {
                w1617 = 0.0
                # "motoren sterk links sneller"
                n195 = xnode "Analog output (1 sample) 37"("A/AO0 (Pin 2)"=w1617) -> ()  [unwired: 1 in, 1 out]
                n196 = xnode "Analog output (1 sample) 39"("B/AO0 (Pin 2)"=w1617) -> ()  [unwired: 1 in, 1 out]
                n197 = xnode "Analog output (1 sample) 38"("A/AO1 (Pin 4)"=5.0) -> ()  [unwired: 1 in, 1 out]
                n198 = xnode "Analog output (1 sample) 40"("B/AO1 (Pin 4)"=2.0) -> ()  [unwired: 1 in, 1 out]
              }
            }
            n199 = case shown="True" w531 {
              frame False {
              }
              frame True {
                w1315 = 0.0
                # "motor naar rechts sneller"
                n200 = xnode "Analog output (1 sample) 41"("A/AO0 (Pin 2)"=w1315) -> ()  [unwired: 1 in, 1 out]
                n201 = xnode "Analog output (1 sample) 43"("B/AO0 (Pin 2)"=w1315) -> ()  [unwired: 1 in, 1 out]
                n202 = xnode "Analog output (1 sample) 44"("B/AO1 (Pin 4)"=5.0) -> ()  [unwired: 1 in, 1 out]
                n203 = xnode "Analog output (1 sample) 42"("A/AO1 (Pin 4)"=3.0) -> ()  [unwired: 1 in, 1 out]
              }
            }
            n204 = case shown="True" w528 {
              frame False {
              }
              frame True {
                w711 = 0.0
                # "motor sterk rechts sneller"
                n205 = xnode "Analog output (1 sample) 47"("B/AO0 (Pin 2)"=w711) -> ()  [unwired: 1 in, 1 out]
                n206 = xnode "Analog output (1 sample) 45"("A/AO0 (Pin 2)"=w711) -> ()  [unwired: 1 in, 1 out]
                n207 = xnode "Analog output (1 sample) 48"("B/AO1 (Pin 4)"=5.0) -> ()  [unwired: 1 in, 1 out]
                n208 = xnode "Analog output (1 sample) 46"("A/AO1 (Pin 4)"=2.0) -> ()  [unwired: 1 in, 1 out]
              }
            }
          }
          frame True {
            # "groen licht FALSE"
            # "rood licht TRUE"
            n209 = global read "Global 1.vi" "Array"() -> (w2112:dbl[])
            n210 = Index Array(array=w2112, index=0) -> (element=w2110:dbl)
            n211 = Equal?(x=1, y=w2110) -> (x = y?=w2115:bool)
            n212 = Equal?(x=w2110, y=2) -> (x = y?=w2114:bool)
            n213 = Equal?(x=w2110, y=3) -> (x = y?=w2113:bool)
            n214 = flat-sequence {
              tunnel: [w2242] -> w2104
              tunnel: [w2241] -> w2103
              frame #0 {
                w2120 = 41 ("Numeric")
                # "154ms"
                # "ID of the RGB-sensor"
                # "Command Register: 100 00000\nCombined with Enable: 0000 0011"
                # "Command Register: 100 01111\nCombined with Control(Gain to x1): 0000 0000"
                # "Command Register: 100 00001\nCombined with Timing: 0000 0000"
                n215 = String To Byte Array(string="€\u0003") -> (unsigned byte array=w2123:u8[])
                n216 = xnode "I2C 3"("Slave Address (7-bit)"=w2120, "Bytes to Write"=w2123, "error in (no error)"="error in (no error) 3") -> ("error out"=w2119:errorcluster)
                n217 = String To Byte Array(string="\u0000") -> (unsigned byte array=w2122:u8[])
                n218 = xnode "I2C 2"("Slave Address (7-bit)"=w2120, "Bytes to Write"=w2122, "error in (no error)"=w2119) -> ("error out"=w2118:errorcluster)
                n219 = String To Byte Array(string="À") -> (unsigned byte array=w2121:u8[])
                n220 = xnode "I2C"("Slave Address (7-bit)"=w2120, "Bytes to Write"=w2121, "error in (no error)"=w2118) -> ("error out"=→"error out 3":errorcluster)
              }
              frame #1 {
                n221 = while {
                  shift-right: [w2259] -> _
                  shift-left: 0 -> [w2261]
                  shift-right: [w2255] -> w2241
                  shift-left: 0 -> [w2257]
                  stop <- w2260 stop-if-true
                  n222 = Increment(x=w2261) -> (x+1=w2259:i32)
                  n223 = Wait (ms)(milliseconds to wait=u32 154) -> ()  [unwired: 1 out]
                  n224 = call "kleursensor.vi"() -> ("Total 2"=w2256:u32)  [unwired: 8 in, 3 out]
                  n225 = Add(x=w2257, y=w2256) -> (x+y=w2255:u32)
                  n226 = Equal?(x=w2259, y=20) -> (x = y?=w2260:bool)
                }
                "rood" <- w2241
                n227 = while {
                  shift-right: [w2251] -> _
                  shift-left: 0 -> [w2253]
                  shift-right: [w2247] -> w2242
                  shift-left: 0 -> [w2248]
                  stop <- w2252 stop-if-true
                  n228 = Increment(x=w2253) -> (x+1=w2251:i32)
                  n229 = Wait (ms)(milliseconds to wait=u32 154) -> ()  [unwired: 1 out]
                  n230 = call "kleursensor2.vi"() -> ("Total"=w2249:u32)  [unwired: 8 in, 3 out]
                  n231 = Add(x=w2248, y=w2249) -> (x+y=w2247:u32)
                  n232 = Equal?(x=w2251, y=20) -> (x = y?=w2252:bool)
                }
                "groen" <- w2242
              }
            }
            n233 = Add(x=w2104, y=50) -> (x+y=w2106:u32)
            n234 = Greater?(x=w2103, y=w2106) -> (0:w2102:bool)
            n235 = case shown="True" w2113 {
              tunnel: w2102 -> [w2263 w2265]
              tunnel: [w2263 w2264] -> w2101
              frame False {
              }
              frame True {
                n236 = flat-sequence {
                  tunnel: w2265 -> [w2417]
                  tunnel: [w2416] -> w2264
                  frame #0 {
                    w2266 = 0.0
                    # "motor  stilleggen"
                    n237 = xnode "Analog output (1 sample) 12"("A/AO0 (Pin 2)"=w2266) -> ()  [unwired: 1 in, 1 out]
                    n238 = xnode "Analog output (1 sample) 57"("A/AO1 (Pin 4)"=w2266) -> ()  [unwired: 1 in, 1 out]
                    n239 = xnode "Analog output (1 sample) 11"("B/AO0 (Pin 2)"=w2266) -> ()  [unwired: 1 in, 1 out]
                    n240 = xnode "Analog output (1 sample) 58"("B/AO1 (Pin 4)"=w2266) -> ()  [unwired: 1 in, 1 out]
                  }
                  frame #1 {
                    n241 = Get Date/Time In Seconds() -> (seconds since 1Jan1904=w2415:timestamp)
                    n242 = while {
                      tunnel: w2417 -> [w2419]
                      tunnel: [w2419] -> w2416
                      tunnel: w2415 -> [w2418]
                      stop <- w2420 stop-if-true
                      # "kleursensor"
                      n243 = case shown="False" w2419 {
                        tunnel: [w2421 FALSE] -> w2420
                        tunnel: w2418 -> [w2422 _]
                        frame False {
                          w2427 = 0.0
                          n244 = Get Date/Time In Seconds() -> (seconds since 1Jan1904=w2423:timestamp)
                          n245 = Subtract(x=w2423, y=w2422) -> (x-y=w2425:dbl)
                          n246 = Greater Or Equal?(x=w2425, y="tijdsinterval 6") -> (x >= y?=w2421:bool)
                          n247 = xnode "Analog output (1 sample) 78"("B/AO0 (Pin 2)"=w2427) -> ()  [unwired: 1 in, 1 out]
                          n248 = xnode "Analog output (1 sample) 76"("A/AO0 (Pin 2)"=w2427) -> ()  [unwired: 1 in, 1 out]
                          n249 = xnode "Analog output (1 sample) 77"("A/AO1 (Pin 4)"=5.0) -> ()  [unwired: 1 in, 1 out]
                          n250 = xnode "Analog output (1 sample) 79"("B/AO1 (Pin 4)"=5.0) -> ()  [unwired: 1 in, 1 out]
                        }
                        frame True {
                        }
                      }
                    }
                  }
                  frame #2 {
                    n251 = Get Date/Time In Seconds() -> (seconds since 1Jan1904=w2578:timestamp)
                    n252 = while {
                      tunnel: w2578 -> [w2579]
                      stop <- w2580 stop-if-true
                      w2585 = 0.0
                      # "rechts 90 graden draaien"
                      n253 = xnode "Analog output (1 sample) 67"("B/AO0 (Pin 2)"=w2585) -> ()  [unwired: 1 in, 1 out]
                      n254 = xnode "Analog output (1 sample) 65"("A/AO0 (Pin 2)"=w2585) -> ()  [unwired: 1 in, 1 out]
                      n255 = Get Date/Time In Seconds() -> (seconds since 1Jan1904=w2583:timestamp)
                      n256 = Subtract(x=w2583, y=w2579) -> (x-y=w2581:dbl)
                      n257 = Greater Or Equal?(x=w2581, y="tijdsinterval 8") -> (x >= y?=w2580:bool)
                      n258 = xnode "Analog output (1 sample) 66"("A/AO1 (Pin 4)"=0.0) -> ()  [unwired: 1 in, 1 out]
                      n259 = xnode "Analog output (1 sample) 68"("B/AO1 (Pin 4)"=5.0) -> ()  [unwired: 1 in, 1 out]
                    }
                  }
                  frame #3 {
                    n260 = Get Date/Time In Seconds() -> (seconds since 1Jan1904=w2735:timestamp)
                    n261 = while {
                      tunnel: w2735 -> [w2737]
                      stop <- w2736 stop-if-true
                      w2742 = 0.0
                      n262 = Get Date/Time In Seconds() -> (seconds since 1Jan1904=w2740:timestamp)
                      n263 = xnode "Analog output (1 sample) 82"("B/AO0 (Pin 2)"=w2742) -> ()  [unwired: 1 in, 1 out]
                      n264 = Subtract(x=w2740, y=w2737) -> (x-y=w2738:dbl)
                      n265 = xnode "Analog output (1 sample) 80"("A/AO0 (Pin 2)"=w2742) -> ()  [unwired: 1 in, 1 out]
                      n266 = Greater Or Equal?(x=w2738, y="tijdsinterval 7") -> (x >= y?=w2736:bool)
                      n267 = xnode "Analog output (1 sample) 81"("A/AO1 (Pin 4)"=5.0) -> ()  [unwired: 1 in, 1 out]
                      n268 = xnode "Analog output (1 sample) 83"("B/AO1 (Pin 4)"=5.0) -> ()  [unwired: 1 in, 1 out]
                    }
                  }
                  frame #4 {
                    n269 = global read "Global 1.vi" "Array"() -> (w2894:dbl[])
                    n270 = Delete From Array(array=w2894, length=1, index=0) -> (array with subset deleted=w2895:dbl[])  [unwired: 1 out]
                    n271 = global write "Global 1.vi" "Array"(w2895) -> ()
                  }
                }
              }
            }
            n272 = case shown="True" w2114 {
              tunnel: w2101 -> [w3525 w3527]
              tunnel: [w3525 w3526] -> w2100
              frame False {
              }
              frame True {
                n273 = flat-sequence {
                  tunnel: w3527 -> [w3679]
                  tunnel: [w3678] -> w3526
                  frame #0 {
                    w3528 = 0.0
                    # "motor  stilleggen"
                    n274 = xnode "Analog output (1 sample) 8"("A/AO0 (Pin 2)"=w3528) -> ()  [unwired: 1 in, 1 out]
                    n275 = xnode "Analog output (1 sample) 56"("B/AO1 (Pin 4)"=w3528) -> ()  [unwired: 1 in, 1 out]
                    n276 = xnode "Analog output (1 sample) 55"("A/AO1 (Pin 4)"=w3528) -> ()  [unwired: 1 in, 1 out]
                    n277 = xnode "Analog output (1 sample) 7"("B/AO0 (Pin 2)"=w3528) -> ()  [unwired: 1 in, 1 out]
                  }
                  frame #1 {
                    n278 = Get Date/Time In Seconds() -> (seconds since 1Jan1904=w3677:timestamp)
                    n279 = while {
                      tunnel: w3679 -> [w3681]
                      tunnel: [w3681] -> w3678
                      tunnel: w3677 -> [w3680]
                      stop <- w3682 stop-if-true
                      # "kleursensor"
                      n280 = case shown="False" w3681 {
                        tunnel: [w3683 FALSE] -> w3682
                        tunnel: w3680 -> [w3684 _]
                        frame False {
                          w3689 = 0.0
                          # "rechtdoor"
                          n281 = Get Date/Time In Seconds() -> (seconds since 1Jan1904=w3687:timestamp)
                          n282 = Subtract(x=w3687, y=w3684) -> (x-y=w3685:dbl)
                          n283 = Greater Or Equal?(x=w3685, y="tijdsinterval 5") -> (x >= y?=w3683:bool)
                          n284 = xnode "Analog output (1 sample) 9"("A/AO0 (Pin 2)"=w3689) -> ()  [unwired: 1 in, 1 out]
                          n285 = xnode "Analog output (1 sample) 63"("B/AO0 (Pin 2)"=w3689) -> ()  [unwired: 1 in, 1 out]
                          n286 = xnode "Analog output (1 sample) 10"("A/AO1 (Pin 4)"=5.0) -> ()  [unwired: 1 in, 1 out]
                          n287 = xnode "Analog output (1 sample) 64"("B/AO1 (Pin 4)"=5.0) -> ()  [unwired: 1 in, 1 out]
                        }
                        frame True {
                        }
                      }
                    }
                  }
                  frame #2 {
                    n288 = global read "Global 1.vi" "Array"() -> (w3842:dbl[])
                    n289 = Delete From Array(array=w3842, length=1, index=0) -> (array with subset deleted=w3843:dbl[])  [unwired: 1 out]
                    n290 = global write "Global 1.vi" "Array"(w3843) -> ()
                  }
                }
              }
            }
            n291 = case shown="True" w2115 {
              tunnel: w2100 -> [_ w2896]
              frame False {
              }
              frame True {
                n292 = flat-sequence {
                  tunnel: w2896 -> [w3047]
                  frame #0 {
                    w2897 = 0.0
                    # "motor  stilleggen"
                    n293 = xnode "Analog output (1 sample) 54"("B/AO1 (Pin 4)"=w2897) -> ()  [unwired: 1 in, 1 out]
                    n294 = xnode "Analog output (1 sample) 53"("A/AO0 (Pin 2)"=w2897) -> ()  [unwired: 1 in, 1 out]
                    n295 = xnode "Analog output (1 sample)"("A/AO1 (Pin 4)"=w2897) -> ()  [unwired: 1 in, 1 out]
                    n296 = xnode "Analog output (1 sample) 2"("B/AO0 (Pin 2)"=w2897) -> ()  [unwired: 1 in, 1 out]
                  }
                  frame #1 {
                    n297 = Get Date/Time In Seconds() -> (seconds since 1Jan1904=w3046:timestamp)
                    n298 = while {
                      tunnel: w3047 -> [w3049]
                      tunnel: w3046 -> [w3048]
                      stop <- w3050 stop-if-true
                      # "kleursensor"
                      n299 = case shown="False" w3049 {
                        tunnel: [w3052 FALSE] -> w3050
                        tunnel: w3048 -> [w3051 _]
                        frame False {
                          w3056 = 5.0
                          w3057 = 0.0
                          n300 = Get Date/Time In Seconds() -> (seconds since 1Jan1904=w3055:timestamp)
                          n301 = Subtract(x=w3055, y=w3051) -> (x-y=w3053:dbl)
                          n302 = Greater Or Equal?(x=w3053, y="tijdsinterval 2") -> (x >= y?=w3052:bool)
                          n303 = xnode "Analog output (1 sample) 4"("A/AO0 (Pin 2)"=w3057) -> ()  [unwired: 1 in, 1 out]
                          n304 = xnode "Analog output (1 sample) 49"("B/AO0 (Pin 2)"=w3057) -> ()  [unwired: 1 in, 1 out]
                          n305 = xnode "Analog output (1 sample) 50"("B/AO1 (Pin 4)"=w3056) -> ()  [unwired: 1 in, 1 out]
                          n306 = xnode "Analog output (1 sample) 13"("A/AO1 (Pin 4)"=w3056) -> ()  [unwired: 1 in, 1 out]
                        }
                        frame True {
                        }
                      }
                    }
                  }
                  frame #2 {
                    n307 = Get Date/Time In Seconds() -> (seconds since 1Jan1904=w3207:timestamp)
                    n308 = while {
                      tunnel: w3207 -> [w3209]
                      stop <- w3208 stop-if-true
                      w3214 = 0.0
                      # "90 graden draaien naar links"
                      n309 = Get Date/Time In Seconds() -> (seconds since 1Jan1904=w3212:timestamp)
                      n310 = Subtract(x=w3212, y=w3209) -> (x-y=w3210:dbl)
                      n311 = Greater Or Equal?(x=w3210, y="tijdsinterval 3") -> (x >= y?=w3208:bool)
                      n312 = xnode "Analog output (1 sample) 61"("B/AO0 (Pin 2)"=w3214) -> ()  [unwired: 1 in, 1 out]
                      n313 = xnode "Analog output (1 sample) 59"("A/AO0 (Pin 2)"=w3214) -> ()  [unwired: 1 in, 1 out]
                      n314 = xnode "Analog output (1 sample) 60"("A/AO1 (Pin 4)"=5.0) -> ()  [unwired: 1 in, 1 out]
                      n315 = xnode "Analog output (1 sample) 62"("B/AO1 (Pin 4)"=0.0) -> ()  [unwired: 1 in, 1 out]
                    }
                  }
                  frame #3 {
                    n316 = Get Date/Time In Seconds() -> (seconds since 1Jan1904=w3364:timestamp)
                    n317 = while {
                      tunnel: w3364 -> [w3366]
                      stop <- w3365 stop-if-true
                      w3371 = 0.0
                      n318 = Get Date/Time In Seconds() -> (seconds since 1Jan1904=w3369:timestamp)
                      n319 = Subtract(x=w3369, y=w3366) -> (x-y=w3367:dbl)
                      n320 = Greater Or Equal?(x=w3367, y="tijdsinterval 4") -> (x >= y?=w3365:bool)
                      n321 = xnode "Analog output (1 sample) 52"("B/AO0 (Pin 2)"=w3371) -> ()  [unwired: 1 in, 1 out]
                      n322 = xnode "Analog output (1 sample) 74"("A/AO0 (Pin 2)"=w3371) -> ()  [unwired: 1 in, 1 out]
                      n323 = xnode "Analog output (1 sample) 73"("A/AO1 (Pin 4)"=5.0) -> ()  [unwired: 1 in, 1 out]
                      n324 = xnode "Analog output (1 sample) 51"("B/AO1 (Pin 4)"=5.0) -> ()  [unwired: 1 in, 1 out]
                    }
                  }
                  frame #4 {
                    n325 = global read "Global 1.vi" "Array"() -> (w3524:dbl[])
                    n326 = Delete From Array(array=w3524, length=1, index=0) -> (array with subset deleted=w3523:dbl[])  [unwired: 1 out]
                    n327 = global write "Global 1.vi" "Array"(w3523) -> ()
                  }
                }
              }
            }
          }
        }
      }
    }
    frame True {
      # "Manueel bedienen"
      n328 = while {
        tunnel: w3844 -> [w3845]
        stop <- w3845 continue-if-true
        n329 = case shown="True" "links draaien achteruit" {
          frame False {
          }
          frame True {
            w4154 = 0.0
            n330 = xnode "Analog output 7"("B/AO0 (Pin 2)"=2.0) -> ()  [unwired: 1 in, 1 out]
            n331 = xnode "Analog output 9"("A/AO0 (Pin 2)"=5.0) -> ()  [unwired: 1 in, 1 out]
            n332 = xnode "Analog output 6"("B/AO1 (Pin 4)"=w4154) -> ()  [unwired: 1 in, 1 out]
            n333 = xnode "Analog output 8"("A/AO1 (Pin 4)"=w4154) -> ()  [unwired: 1 in, 1 out]
          }
        }
        n334 = case shown="True" "voorwaarts" {
          tunnel: "snelheid" -> [_ w4758]
          frame False {
          }
          frame True {
            w4757 = 0.0
            n335 = xnode "Analog output (1 sample) 16"("A/AO0 (Pin 2)"=w4757) -> ()  [unwired: 1 in, 1 out]
            n336 = xnode "Analog output (1 sample) 15"("B/AO0 (Pin 2)"=w4757) -> ()  [unwired: 1 in, 1 out]
            n337 = xnode "Analog output 3"("A/AO1 (Pin 4)"=w4758) -> ()  [unwired: 1 in, 1 out]
            n338 = xnode "Analog output 2"("B/AO1 (Pin 4)"=w4758) -> ()  [unwired: 1 in, 1 out]
          }
        }
        n339 = case shown="True" "links draaien" {
          frame False {
          }
          frame True {
            w4458 = 0.0
            n340 = xnode "Analog output  rechts 3"("B/AO0 (Pin 2)"=w4458) -> ()  [unwired: 1 in, 1 out]
            n341 = xnode "Analog output  links 2"("A/AO0 (Pin 2)"=w4458) -> ()  [unwired: 1 in, 1 out]
            n342 = xnode "Analog output  rechts 4"("B/AO1 (Pin 4)"=2.0) -> ()  [unwired: 1 in, 1 out]
            n343 = xnode "Analog output  rechts 2"("A/AO1 (Pin 4)"=5.0) -> ()  [unwired: 1 in, 1 out]
          }
        }
        n344 = case shown="True" "stoppen" {
          frame False {
          }
          frame True {
            w3854 = 0.0
            n345 = xnode "Analog output 17"("A/AO0 (Pin 2)"=w3854) -> ()  [unwired: 1 in, 1 out]
            n346 = xnode "Analog output 15"("B/AO0 (Pin 2)"=w3854) -> ()  [unwired: 1 in, 1 out]
            n347 = xnode "Analog output 14"("B/AO1 (Pin 4)"=w3854) -> ()  [unwired: 1 in, 1 out]
            n348 = xnode "Analog output 16"("A/AO1 (Pin 4)"=w3854) -> ()  [unwired: 1 in, 1 out]
          }
        }
        n349 = case shown="True" "achterwaarts" {
          tunnel: "snelheid" -> [_ w4607]
          frame False {
          }
          frame True {
            w4608 = 0.0
            n350 = xnode "Analog output (1 sample) 18"("A/AO0 (Pin 2)"=w4607) -> ()  [unwired: 1 in, 1 out]
            n351 = xnode "Analog output 4"("B/AO0 (Pin 2)"=w4607) -> ()  [unwired: 1 in, 1 out]
            n352 = xnode "Analog output (1 sample) 17"("A/AO1 (Pin 4)"=w4608) -> ()  [unwired: 1 in, 1 out]
            n353 = xnode "Analog output 5"("B/AO1 (Pin 4)"=w4608) -> ()  [unwired: 1 in, 1 out]
          }
        }
        n354 = case shown="True" "rechts draaien achteruit" {
          frame False {
          }
          frame True {
            w4004 = 0.0
            n355 = xnode "Analog output 13"("A/AO0 (Pin 2)"=2.0) -> ()  [unwired: 1 in, 1 out]
            n356 = xnode "Analog output 11"("B/AO0 (Pin 2)"=5.0) -> ()  [unwired: 1 in, 1 out]
            n357 = xnode "Analog output 10"("B/AO1 (Pin 4)"=w4004) -> ()  [unwired: 1 in, 1 out]
            n358 = xnode "Analog output 12"("A/AO1 (Pin 4)"=w4004) -> ()  [unwired: 1 in, 1 out]
          }
        }
        n359 = case shown="True" "rechts draaien" {
          frame False {
          }
          frame True {
            w4307 = 0.0
            n360 = xnode "Analog output  rechts 5"("B/AO0 (Pin 2)"=w4307) -> ()  [unwired: 1 in, 1 out]
            n361 = xnode "Analog output  links"("A/AO0 (Pin 2)"=w4307) -> ()  [unwired: 1 in, 1 out]
            n362 = xnode "Analog output  rechts 6"("B/AO1 (Pin 4)"=5.0) -> ()  [unwired: 1 in, 1 out]
            n363 = xnode "Analog output  rechts"("A/AO1 (Pin 4)"=2.0) -> ()  [unwired: 1 in, 1 out]
          }
        }
      }
    }
  }
